vi "h.COMM.Execute Command.vi"(0 "Connection ID":refnum<k5>, 5 "Command":string, 7 "Timeout":i32=10000, 9 "Argument":string, 11 "error in":errorcluster) -> (1 "Content":u8[](array[numeric]), 3 "Status":T2, 4 "Connection ID out":refnum<k5>, 6 "Request Option Echo":T1=enum."Suppress Message", 8 "Message Length":u16, 10 "Message":string, 13 "Content Length":u32, 15 "error out":errorcluster)   [LabVIEW 2019, in "h.Library.lvlib"]
doc: "This vi executes a Hyperion command and reports the result and any data returned by the command.\n\n<b>Connection ID</b> - is a network connection refnum that uniquely identifies the TCP connection\n<b>Command</b> - Hyperion command to execute\n<b>Command Content</b> - arguments to the command\n<b>Timeout</b> - specifies the maximum amount of time, in milliseconds, for the function to complete\n<b>error in</b> - describes error conditions that occur before this node runs. This input provides standard error functionality\n<b>Connection ID out</b> - returns the same value as connection ID\n<b>Status</b> - status of the executed command \n<b>Content</b> - data optionally returned by the executed command\n<b>Content Length</b> - byte-length of <b>Content</b>\n<b>Type</b> - response type\n<b>Message</b> - human readable string reporting the outcome of the executed command\n<b>Message Length</b> - byte-length of <b>Message</b>\n<b>error out</b> - contains error information. This output provides standard error out functionality."
uses:
  h.Library.lvlib
  CTL/h.COMM.Command Status Enum.ctl
  CTL/h.COMM.RequestCommandOptions.ctl
panel:
  out "Elapsed Time":dbl
  # "Hyperion Execute Command"
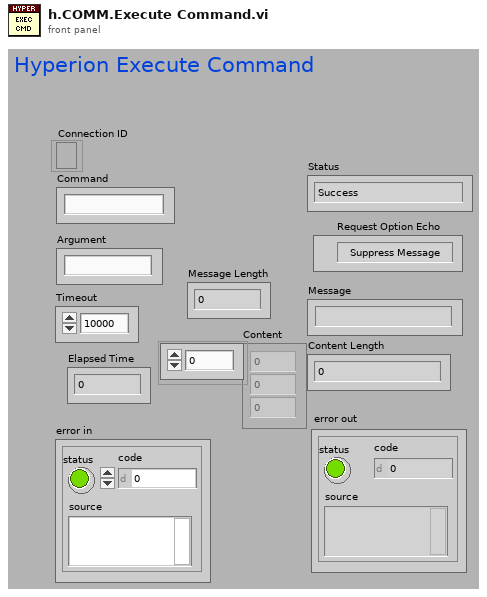
[diagram p1: front panel]
types:
  T1 = typedef "h.Library.lvlib/h.COMM.RequestCommandOptions.ctl" = enum8{"None", "Suppress Message", "Suppress Content", "Compress"}
  T2 = typedef "h.Library.lvlib/h.COMM.Command Status Enum.ctl" = enum8{"Success", "Failed", "Error", "AccessDenied", "InvalidCommand", "InvalidNumberArguments", "InvalidArgument", ""}
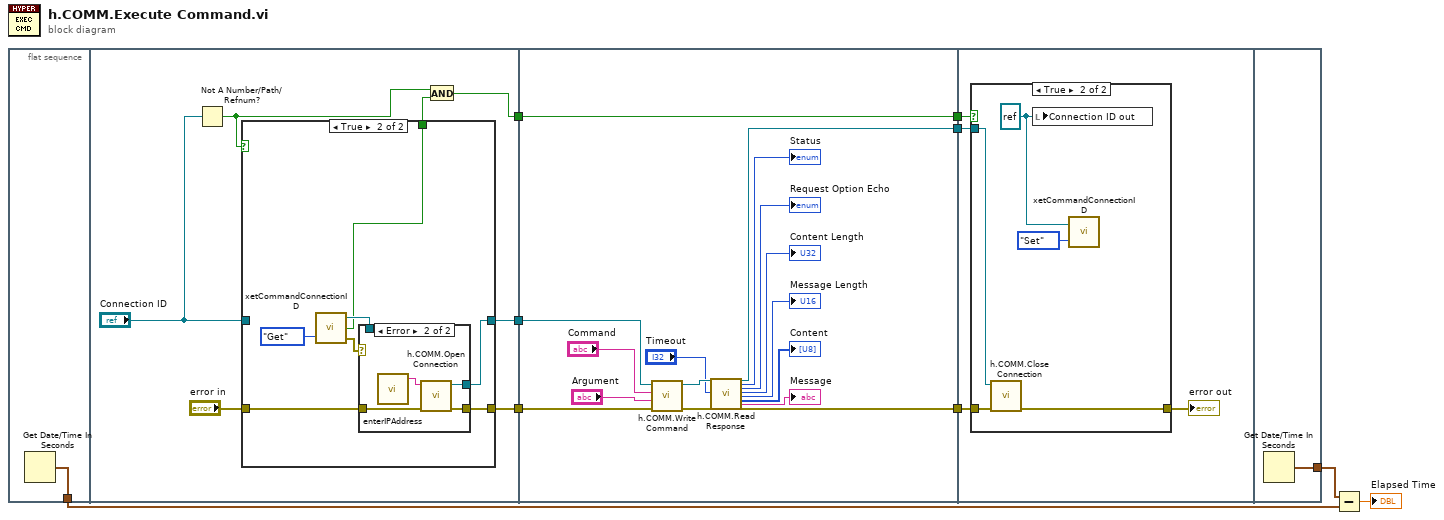
[diagram p0: block diagram]
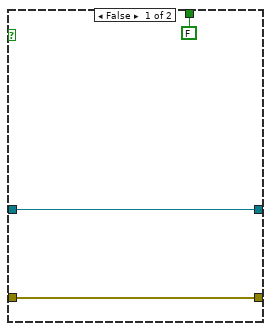
[diagram p2: hidden frame]
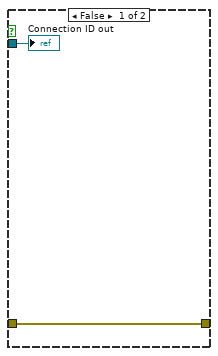
[diagram p4: hidden frame]
diagram:
  n1 = flat-sequence {
    tunnel: [w10] -> w8
    tunnel: [w17] -> w6
    tunnel: [w11] -> w4
    tunnel: [w15] -> w1
    tunnel: w6 -> [w38]
    tunnel: [w37] -> w5
    tunnel: w4 -> [w37]
    tunnel: [w36] -> w3
    tunnel: [w35] -> w2
    tunnel: w1 -> [w34]
    tunnel: w5 -> [w53]
    tunnel: w3 -> [w52]
    tunnel: w2 -> [w51]
    tunnel: [w61] -> w9
    frame #0 {
      n2 = Get Date/Time In Seconds() -> (seconds since 1Jan1904=w10:timestamp)
    }
    frame #1 {
      n3 = Not A Number/Path/Refnum?(number/path/refnum="Connection ID") -> (NaN/Path/Refnum?=w12:bool)
      n4 = case shown="True" w12 {
        tunnel: [w20 w22] -> w17
        tunnel: "Connection ID" -> [w20 _]
        tunnel: [w19 w25] -> w15
        tunnel: "error in" -> [w19 w24]
        tunnel: [FALSE ("New Connection") w21] -> w13
        frame False {
        }
        frame True {
          n5 = call "xetCommandConnectionID.vi"("Get/Set"=enum16{"Get", "Set"}."Get") -> ("Connection ID Out"=w23:refnum<k5>, "New Connection"=w21:bool, "error out"=w26:errorcluster)  [unwired: 2 in]
          n6 = case shown="Error" w26 {
            tunnel: w24 -> [w29 w32]
            tunnel: [w29 w31] -> w25
            tunnel: w23 -> [w28 _]
            tunnel: [w28 w30] -> w22
            frame No Error {
            }
            frame Error {
              n7 = call "enterIPAddress.vi"() -> ("IP Address Out"=w33:string)  [unwired: 2 in, 1 out]
              n8 = call "h.COMM.Open Connection.vi"("error in"=w32, "Address"=w33) -> ("error out"=w31:errorcluster, "Connection ID"=w30:refnum<k5>)  [unwired: 8 in]
            }
          }
        }
      }
      n9 = And(x=w12, y=w13) -> (x .and. y?=w11:bool)
    }
    frame #2 {
      n10 = call "h.COMM.Write Command.vi"("error in"=w34, "Argument"="Argument", "Command"="Command", "Connection ID"=w38) -> ("error out"=w39:errorcluster, "Connection ID out"=w47:refnum<k5>)  [unwired: 6 in]
      n11 = call "h.COMM.Read Response.vi"("Connection ID"=w47, "Timeout"="Timeout", "error in"=w39) -> ("Connection ID"=w36:refnum<k5>, "Status"=→"Status":T2, "Request Option Echo"=→"Request Option Echo":T1, "Content Length"=→"Content Length":u32, "Message Length"=→"Message Length":u16, "Content"=→"Content":u8[], "Message"=→"Message":string, "error out"=w35:errorcluster)  [unwired: 17 in]
    }
    frame #3 {
      n12 = case shown="True" w53 {
        tunnel: w52 -> [w55 w58]
        tunnel: w51 -> [w54 w60]
        tunnel: [w54 w59] -> w50
        frame False {
          "Connection ID out" <- w55
        }
        frame True {
          w57 = refnum<k5> refnum ("Connection ID out")
          n13 = call "h.COMM.Close Connection.vi"("error in"=w60, "Connection ID"=w58) -> ("error out"=w59:errorcluster)  [unwired: 9 in]
          n14 = local write "Connection ID out"(w57) -> ()
          n15 = call "xetCommandConnectionID.vi"("Connection ID In"=w57, "Get/Set"=enum16{"Get", "Set"}."Set") -> ()  [unwired: 1 in, 3 out]
        }
      }
      "error out" <- w50
    }
    frame #4 {
      n16 = Get Date/Time In Seconds() -> (seconds since 1Jan1904=w61:timestamp)
    }
  }
  n17 = Subtract(x=w9, y=w8) -> (x-y=→"Elapsed Time":dbl)
